vi "MeasureVoltage.vi"(8 "error in (no error)":errorcluster, 11 "Keysight in":refnum<class "Keysight.lvclass">) -> (0 "error out":errorcluster, 3 "Keysight out":refnum<class "Keysight.lvclass">)   [LabVIEW 2020, in "Keysight.lvclass"]
uses:
  Keysight/Keysight.lvclass
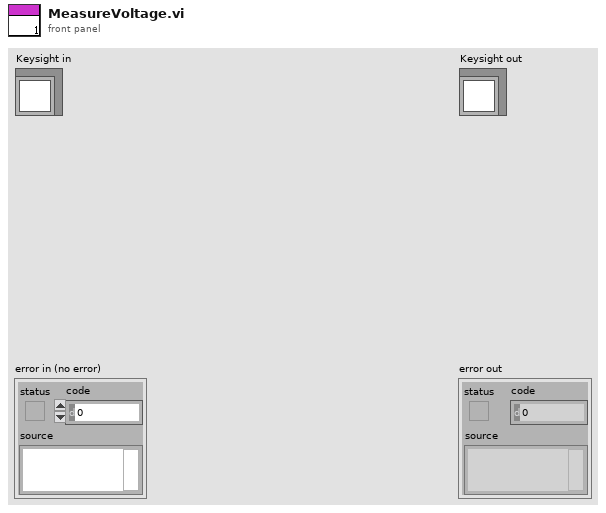
[diagram p1: front panel]
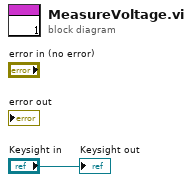
[diagram p0: block diagram]
diagram:
  "Keysight out" <- "Keysight in"
